vi "Swerve Wheel 2020.vi"(0 "Wheelbase Length":dbl=28.0, 5 "Wheelbase Width":dbl=27.5) -> ()   [LabVIEW 2018]
uses:
  Robot Global Data.vi
  <vilib>/Rock Robotics/WPI/ThirdParty/Phoenix-LabVIEW/Motor Controller/Get/CTRE_Phoenix_MotorController_GetSelectedSensorData.vi
panel:
  out "Wheel Loop Speed":u32=31
  in  "Rot. Point X":dbl
  in  "Rot. Point Y":dbl
  # "SWERVE Wheel 2020\nVersion 2020\nStudent Contributors over the years:\nCory Lynch\nChris Garuti\nGavin Popkin\nKaitlyn Sandor\nEthan Silver\nApple Pi Robotics\nTeam 2067"
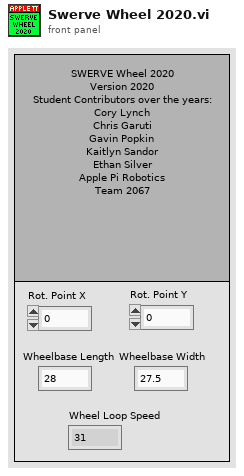
[diagram p1: front panel]
types:
  T1 = typedef "WPI_MotorControlDeviceRef.ctl" = cluster{"DeviceStatus":errorcluster, "Type":T2, "PWM":cluster{"PWM Channel":T3, "DeadBand":T4}, "CAN":cluster{"Device Number":u8, "SetOutput VI Ref":variant, "GetOutput VI Ref":variant, "Enable VI Ref":variant, "Disable VI Ref":variant, "Data":variant}, "Invert":bool, "DIO PWM":cluster{"PWM \"Enable\" Channel":T3, "DIOChannel":T5, "PWM Rate":dbl}}
  T2 = typedef "WPI_MotorControlType.ctl" = enum16{"PWM", "CAN", "DIO PWM"}
  T3 = typedef "FPGA_DIOPWMChannel.ctl" = enum8{"PWM 0", "PWM 1", "PWM 2", "PWM 3", "PWM 4", "PWM 5", "PWM 6", "PWM 7", "PWM 8", "PWM 9", "PWM MXP 0", "PWM MXP 1", "PWM MXP 2", "PWM MXP 3", "PWM MXP 4", "PWM MXP 5", "PWM MXP 6", "PWM MXP 7", "PWM MXP 8", "PWM MXP 9", "Invalid"}
  T4 = typedef "WPI_PWMDeadband.ctl" = cluster{"Name":string, "maxPositivePwm":i32, "minPositivePwm":i32, "centerPwm":i32, "maxNegativePwm":i32, "minNegativePwm":i32, "angularRange":u16}
  T5 = typedef "FPGA_DIOChannel.ctl" = enum8{"DIO 0", "DIO 1", "DIO 2", "DIO 3", "DIO 4", "DIO 5", "DIO 6", "DIO 7", "DIO 8", "DIO 9", "DIO MXP 0", "DIO MXP 1", "DIO MXP 2", "DIO MXP 3", "DIO MXP 4", "DIO MXP 5", "DIO MXP 6", "DIO MXP 7", "DIO MXP 8", "DIO MXP 9", "DIO MXP 10", "DIO MXP 11", "DIO MXP 12", "DIO MXP 13", "DIO MXP 14", "DIO MXP 15", "SPI Port CS1", "SPI Port CS2", "SPI Port CS3", "SPI Port MISO", "SPI Port MOSI", "Invalid"}
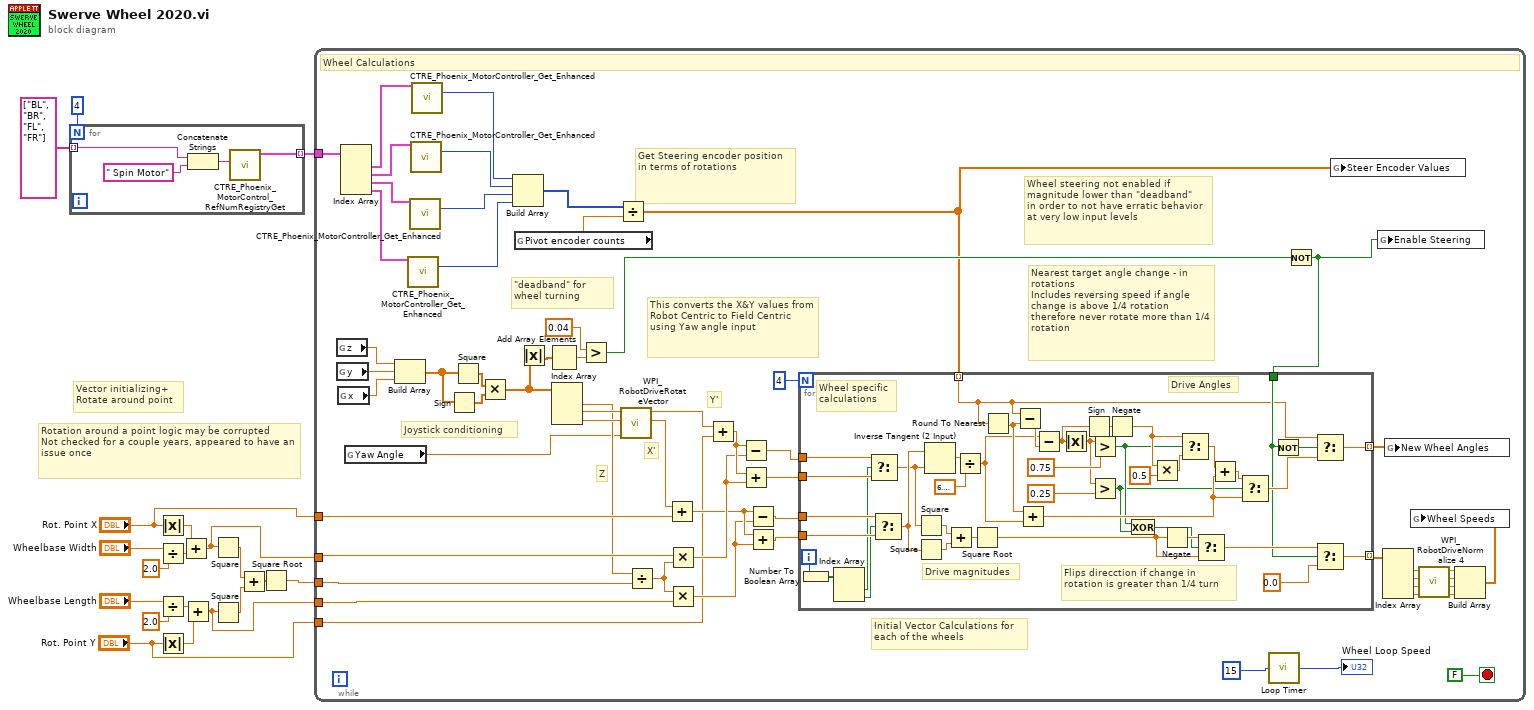
[diagram p0: block diagram]
diagram:
  # "Rotation around a point logic may be corrupted\nNot checked for a couple years, appeared to have an issue once"
  # "Vector initializing+\nRotate around point"
  n1 = for {
    N: 4 -> [_]
    tunnel: string[] ["BL", "BR", "FL", "FR"] -> [w23] mode=indexing
    tunnel: [w20] -> w2 mode=indexing
    n2 = Concatenate Strings(w23, " Spin Motor" ("refnum name")) -> (w22:string)
    n3 = call <vilib>:"CTRE_Phoenix_MotorControl_RefNumRegistryGet.vi"("refnum name"=w22) -> ("PhoenixMotorControlDevRef"=w20:T1)  [unwired: 9 in, 1 out]
  }
  n4 = Absolute Value(x="Rot. Point X") -> (abs(x)=w5:dbl)
  n5 = Divide(x="Wheelbase Width", y=2.0) -> (x/y=w15:dbl)
  n6 = Divide(x="Wheelbase Length", y=2.0) -> (x/y=w16:dbl)
  n7 = Absolute Value(x="Rot. Point Y") -> (abs(x)=w17:dbl)
  n8 = Add(x=w5, y=w15) -> (x+y=w7:dbl)
  n9 = Add(x=w16, y=w17) -> (x+y=w4:dbl)
  n10 = Square(x=w7) -> (x^2=w12:dbl)
  n11 = Square(x=w4) -> (x^2=w13:dbl)
  n12 = Add(x=w12, y=w13) -> (x+y=w11:dbl)
  n13 = Square Root(x=w11) -> (sqrt(x)=w6:dbl)
  n14 = while {
    tunnel: w7 -> [w60]
    tunnel: "Rot. Point X" -> [w59]
    tunnel: w4 -> [w58]
    tunnel: w6 -> [w57]
    tunnel: "Rot. Point Y" -> [w56]
    tunnel: w2 -> [w34]
    stop <- FALSE stop-if-true
    # "Wheel steering not enabled if \nmagnitude lower than \"deadband\"\nin order to not have erratic behavior at very low input levels"
    # "Z"
    # "X'"
    # "Y'"
    # "\"deadband\" for wheel turning"
    # "Joystick conditioning"
    # "Get Steering encoder position in terms of rotations"
    # "This converts the X&Y values from Robot Centric to Field Centric using Yaw angle input"
    # "Nearest target angle change - in rotations\nIncludes reversing speed if angle change is above 1/4 rotation\ntherefore never rotate more than 1/4 rotation"
    # "Initial Vector Calculations for\neach of the wheels"
    # "Wheel Calculations"
    n15 = global read "Robot Global Data.vi" "z"() -> (w26:dbl)
    n16 = global read "Robot Global Data.vi" "y"() -> (w45:dbl)
    n17 = global read "Robot Global Data.vi" "x"() -> (w44:dbl)
    n18 = Index Array(array=w34) -> (element #1=w38:T1, element #2=w37:T1, element #3=w36:T1, element #4=w35:T1)  [unwired: 4 in]
    n19 = global read "Robot Global Data.vi" "Yaw Angle"() -> (w30:dbl)
    n20 = Build Array(w26, w45, w44) -> (w43:dbl[])
    n21 = call-poly <vilib>:"CTRE_Phoenix_MotorController_Get_Enhanced.vi"("PhoenixMotorControlDevRef"=w35) -> ("Position (Raw Sensor Units)"=w54:i32)  [unwired: 11 in, 3 out]
    n22 = call-poly <vilib>:"CTRE_Phoenix_MotorController_Get_Enhanced.vi"("PhoenixMotorControlDevRef"=w36) -> ("Position (Raw Sensor Units)"=w55:i32)  [unwired: 11 in, 3 out]
    n23 = call-poly <vilib>:"CTRE_Phoenix_MotorController_Get_Enhanced.vi"("PhoenixMotorControlDevRef"=w37) -> ("Position (Raw Sensor Units)"=w53:i32)  [unwired: 11 in, 3 out]
    n24 = call-poly <vilib>:"CTRE_Phoenix_MotorController_Get_Enhanced.vi"("PhoenixMotorControlDevRef"=w38) -> ("Position (Raw Sensor Units)"=w40:i32)  [unwired: 11 in, 3 out]
    n25 = Sign(1:w43) -> (0:w47:dbl[])
    n26 = Square(x=w43) -> (x^2=w46:dbl[])
    n27 = Multiply(x=w46, y=w47) -> (x*y=w42:dbl[])
    n28 = Build Array(w40, w53, w55, w54) -> (w39:i32[])
    n29 = global read "Robot Global Data.vi" "Pivot encoder counts"() -> (w24:dbl)
    n30 = Absolute Value(x=w42) -> (abs(x)=w48:dbl[])
    n31 = Add Array Elements(numeric array=w48) -> (sum=w50:dbl)
    n32 = Index Array(array=w42) -> (element #1=w41:dbl, element #2=w51:dbl, element #3=w52:dbl)  [unwired: 3 in]
    n33 = Greater?(x=0.04 ("f"), y=w50) -> (0:w33:bool)
    n34 = Divide(x=w39, y=w24) -> (x/y=w29:dbl[])
    n35 = call <vilib>:"WPI_RobotDriveRotateVector.vi"("Angle"=w30, "X"=w52, "Y"=w51) -> ("X'"=w74:dbl, "Y'"=w81:dbl)  [unwired: 7 out]
    n36 = Divide(x=w41, y=w57) -> (x/y=w82:dbl)
    n37 = Add(x=w74, y=w59) -> (x+y=w76:dbl)
    n38 = Multiply(x=w60, y=w82) -> (x*y=w79:dbl)
    n39 = Multiply(x=w82, y=w58) -> (x*y=w75:dbl)
    n40 = Add(x=w81, y=w56) -> (x+y=w80:dbl)
    n41 = Subtract(x=w80, y=w79) -> (x-y=w78:dbl)
    n42 = Add(x=w80, y=w79) -> (x+y=w77:dbl)
    n43 = Subtract(x=w76, y=w75) -> (x-y=w73:dbl)
    n44 = Add(x=w76, y=w75) -> (x+y=w72:dbl)
    n45 = call "Loop Timer.vi"("Wait time"=u32 15 ("millisecond multiple")) -> ("Loop Time"=→"Wheel Loop Speed":u32)
    n46 = Not(x=w33) -> (.not. x?=w25:bool)
    n47 = for {
      N: 4 -> [_]
      tunnel: [w89] -> w71 mode=indexing
      tunnel: w78 -> [w113]
      tunnel: w77 -> [w114]
      tunnel: w73 -> [w116]
      tunnel: w72 -> [w115]
      tunnel: w25 -> [w87]
      tunnel: [w90] -> w32 mode=indexing
      tunnel: w29 -> [w85] mode=indexing
      i -> [w118]
      # "Flips direcction if change in rotation is greater than 1/4 turn"
      # "Drive Angles"
      # "Drive magnitudes"
      # "Wheel specific\ncalculations"
      n48 = Number To Boolean Array(number=w118) -> (Boolean array=w117:bool[])
      n49 = Index Array(array=w117) -> (element #1=w112:bool, element #2=w111:bool)  [unwired: 2 in]
      n50 = Select(t=w113, s=w112, f=w114) -> (s? t:f=w109:dbl)
      n51 = Select(t=w116, s=w111, f=w115) -> (s? t:f=w110:dbl)
      n52 = Square(x=w109) -> (x^2=w123:dbl)
      n53 = Square(x=w110) -> (x^2=w124:dbl)
      n54 = Inverse Tangent (2 Input)(1:w109, 2:w110) -> (0:w119:dbl)
      n55 = Add(x=w123, y=w124) -> (x+y=w122:dbl)
      n56 = Divide(x=w119, y=6.283185307179586) -> (x/y=w102:dbl)
      n57 = Square Root(x=w122) -> (sqrt(x)=w121:dbl)
      n58 = Round To Nearest(number=w85) -> (nearest integer value=w103:dbl)
      n59 = Subtract(x=w85, y=w103) -> (x-y=w108:dbl)
      n60 = Add(x=w103, y=w102) -> (x+y=w98:dbl)
      n61 = Subtract(x=w102, y=w108) -> (x-y=w104:dbl)
      n62 = Absolute Value(x=w104) -> (abs(x)=w106:dbl)
      n63 = Sign(1:w104) -> (0:w100:dbl)
      n64 = Greater?(x=w106, y=0.75) -> (0:w96:bool)
      n65 = Greater?(x=w106, y=0.25) -> (0:w95:bool)
      n66 = Negate(x=w100) -> (-x=w97:dbl)
      n67 = Exclusive Or(1:w95, 2:w96) -> (0:w84:bool)
      n68 = Multiply(x=w97, y=0.5) -> (x*y=w94:dbl)
      n69 = Negate(x=w121) -> (-x=w92:dbl)
      n70 = Select(t=w97, s=w96, f=w94) -> (s? t:f=w99:dbl)
      n71 = Select(t=w92, s=w84, f=w121) -> (s? t:f=w88:dbl)
      n72 = Add(x=w99, y=w98) -> (x+y=w93:dbl)
      n73 = Select(t=w93, s=w95, f=w98) -> (s? t:f=w91:dbl)
      n74 = Not(x=w87) -> (.not. x?=w83:bool)
      n75 = Select(t=w85, s=w83, f=w91) -> (s? t:f=w90:dbl)
      n76 = Select(t=w88, s=w87, f=0.0) -> (s? t:f=w89:dbl)
    }
    n77 = global write "Robot Global Data.vi" "Steer Encoder Values"(w29) -> ()
    n78 = global write "Robot Global Data.vi" "Enable Steering"(w25) -> ()
    n79 = Index Array(array=w71) -> (element #1=w70:dbl, element #2=w69:dbl, element #3=w68:dbl, element #4=w67:dbl)  [unwired: 4 in]
    n80 = global write "Robot Global Data.vi" "New Wheel Angles"(w32) -> ()
    n81 = call <vilib>:"WPI_RobotDriveNormalize 4.vi"("D"=w67, "C"=w68, "B"=w69, "A"=w70) -> ("D'"=w62:dbl, "C'"=w63:dbl, "B'"=w64:dbl, "A'"=w65:dbl)
    n82 = Build Array ("Wheel Speeds")(w65, w64, w63, w62) -> (w31:dbl[])
    n83 = global write "Robot Global Data.vi" "Wheel Speeds"(w31) -> ()
  }
